vi "CoherenceLength.vi"() -> ()   [LabVIEW 2020]
uses:
  C:/Users/quic2/Desktop/DirectUQDLabviewCode/Kinesis/Thorlabs.MotionControl.Controls.dll
  Kinesis/Thorlabs.MotionControl.Controls.dll
  C:/Program Files/Dotfast Consulting/Timetag Explorer 2.26/ttInterface.dll
  Program Files/Dotfast Consulting/Timetag Explorer 2.26/ttInterface.dll
  C:/Users/quic2/Desktop/DirectUQDLabviewCode/Kinesis/Thorlabs.MotionControl.TCube.StepperMotorCLI.dll
  Kinesis/Thorlabs.MotionControl.TCube.StepperMotorCLI.dll
  <vilib>/Utility/file.llb/Write Delimited Spreadsheet (string).vi
  <vilib>/Utility/file.llb/Write Delimited Spreadsheet (I64).vi
  <vilib>/gmath/statdist.llb/st_Percentiles (scalar).vi
  <vilib>/Utility/file.llb/Write Delimited Spreadsheet (DBL).vi
  <vilib>/gmath/NI_Gmath.lvlib
  <vilib>/Analysis/NI_AALBase.lvlib
panel:
  out "Position":dbl
  out "Pos":i32
  in  "Step(mm)":dbl=0.1
  in  "Stop":dbl=5.5
  in  "Start":dbl=4.5
  in  "TCubeStepperControl":refnum<k24>(container)
  out "XY Graph":cluster{dbl[], dbl[]}[](graph)
  out "BG":dbl[](graph)
  out "bVis":dbl
  out "bMin":dbl
  out "bMax":dbl
  out "Ch C Rate":dbl
  out "Ch C":i32
  out "BG Coincidence Rate":dbl
  out "BG Coincidence":i32
  out "Ch C delay UQD unit":i32
  in  "chC delay":dbl=82.8
  in  "Ch C":i32=8
  in  "stop":bool
  out "sVis":dbl
  out "sMin":dbl
  out "sMax":dbl
  out "cVis":dbl
  out "cMin":dbl
  out "cMax":dbl
  out "Singles":dbl[](graph)
  out "Coincidence":dbl[](graph)
  in  "fileName":string="CTW1ns_ACQ_100ms_Rep_100_ITER_2_Scan_50mHz_6V"
  in  "Folder":path=path "D:/PCC/2021/3_March/20thMarch/SinglePhoton/SourceCharacterisation/CoherenceLength/FinalTestCode"
  out "ChB Delay (uqd Unit)":i32
  out "ChADelay(uqd Unit)":i32
  in  "chB delay (ns)":dbl=7.8
  in  "chA delay(ns)":dbl=110.0
  in  "Ch B":u8=7 min=1 max=16 step=1
  in  "Ch A":u8=5 min=1 max=16 step=1
  in  "CTW in ns":dbl=1.0
  out "Peak Coincidence Rate":dbl format="%#_4p"
  out "ChB Rate":dbl format="%#_4p"
  out "ChARate":dbl format="%#_4p"
  out "Peak Coincidence":i32
  out "Ch A":i32
  out "GetTimeCounter":i32
  out "Ch B":i32
  out "GetResolution":dbl
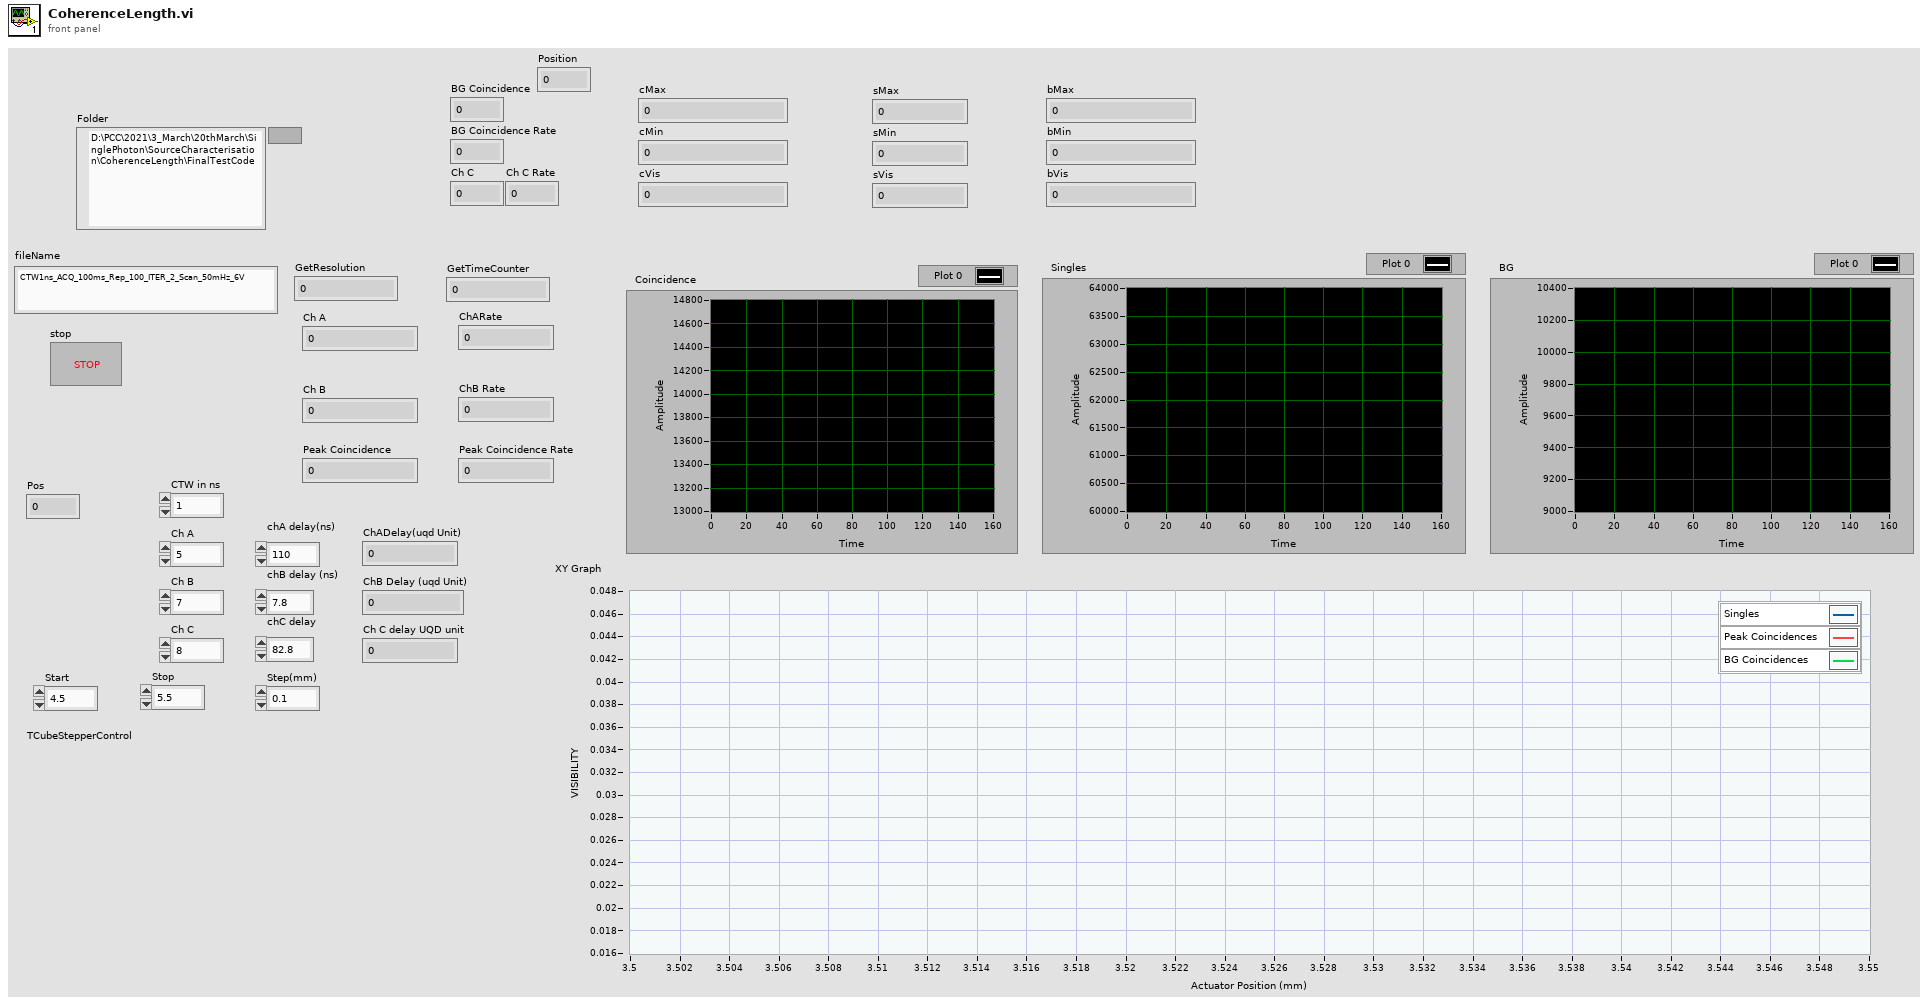
[diagram p1: front panel]
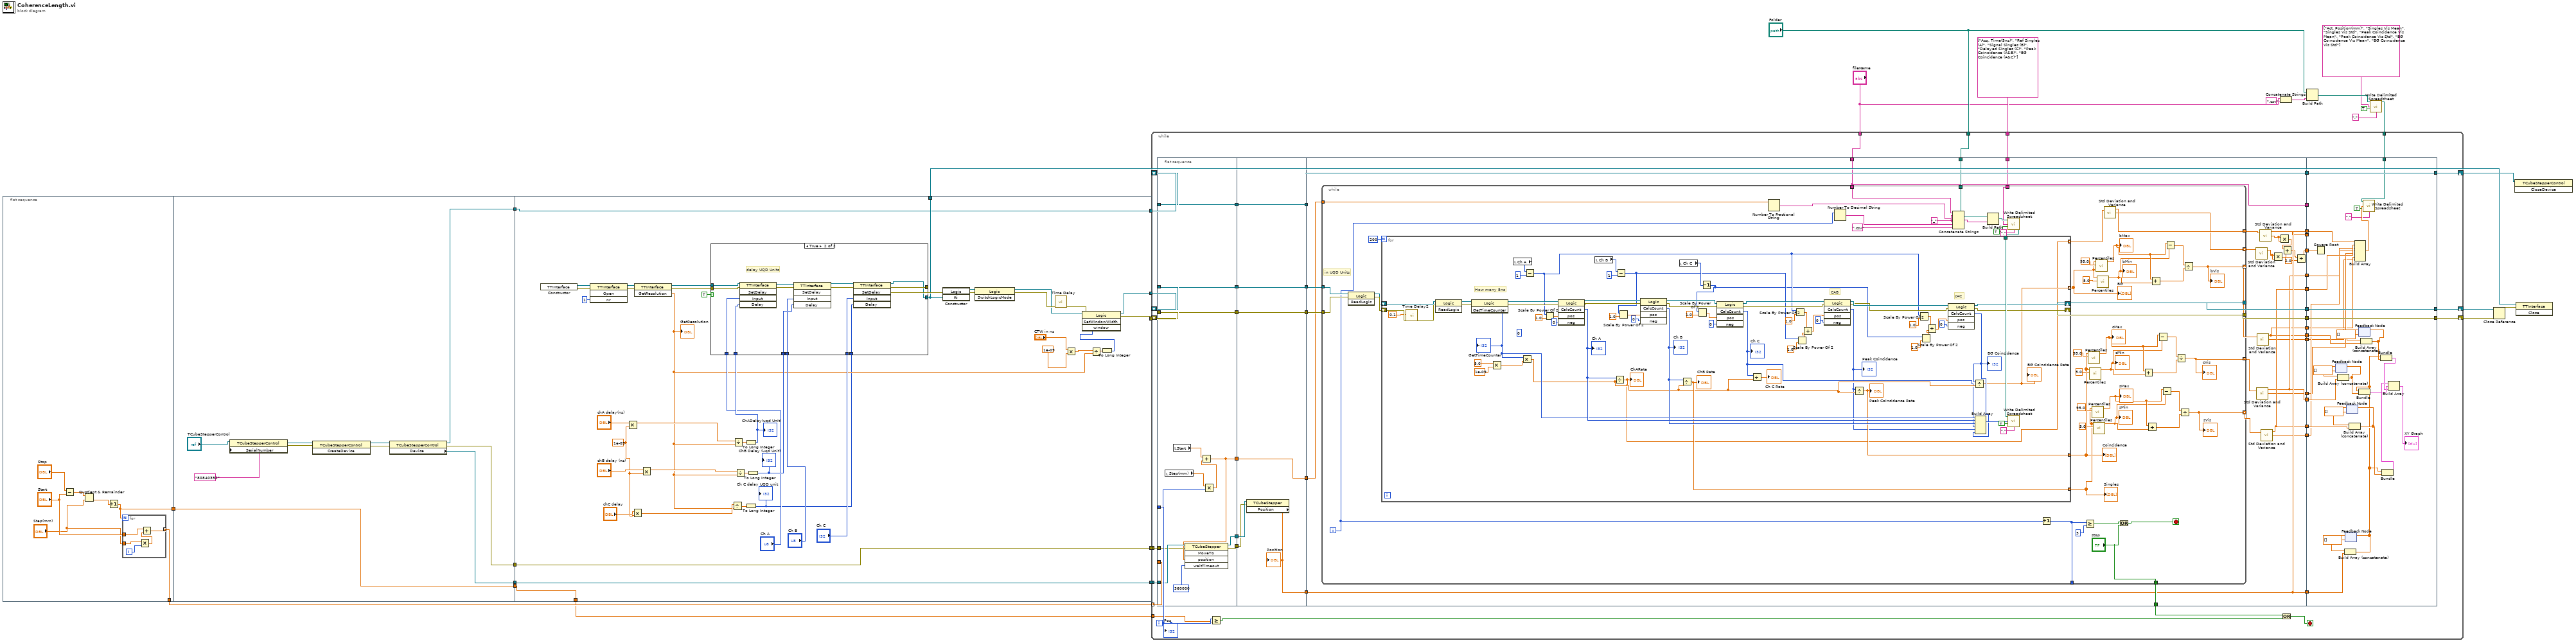
[diagram p0: block diagram]
diagram:
  n1 = flat-sequence {
    tunnel: [w29] -> w14
    tunnel: [w28] -> w11
    tunnel: [w43] -> w21
    tunnel: [w42] -> w20
    tunnel: [w41] -> w16
    tunnel: [w40] -> w12
    tunnel: w11 -> [w40]
    tunnel: [w82] -> w27
    tunnel: [w66] -> w26
    tunnel: [w65] -> w25
    tunnel: w21 -> [w52]
    tunnel: w20 -> [w53]
    tunnel: [w53] -> w19
    tunnel: [w52] -> w17
    tunnel: w16 -> [w51]
    tunnel: [w51] -> w15
    tunnel: [w50] -> w13
    tunnel: w12 -> [w50]
    frame #0 {
      n2 = Subtract(x="Stop", y="Start") -> (x-y=w33:dbl)
      n3 = Quotient & Remainder(x=w33, y="Step(mm)") -> (floor(x/y)=w32:dbl)  [unwired: 1 out]
      n4 = Increment(x=w32) -> (x+1=w28:dbl)
      n5 = for {
        N: w28 -> [_]
        tunnel: "Start" -> [w39]
        tunnel: "Step(mm)" -> [w37]
        tunnel: [w35] -> w29 mode=indexing
        i -> [w38]
        n6 = Multiply(x=w37, y=w38) -> (x*y=w36:dbl)
        n7 = Add(x=w39, y=w36) -> (x+y=w35:dbl)
      }
    }
    frame #1 {
      n8 = property class="TCubeStepperControl"(reference="TCubeStepperControl", "SerialNumber"="80840392") -> (reference out=w46:refnum<k24>, error out=w47:errorcluster)  [unwired: 1 in]
      n9 = invoke class="TCubeStepperControl" method="CreateDevice"(reference=w46, error in=w47) -> (reference out=w45:refnum<k24>, error out=w44:errorcluster)  [unwired: 1 in, 1 out]
      n10 = property class="TCubeStepperControl"(reference=w45, error in=w44) -> (reference out=w42:refnum<k24>, error out=w41:errorcluster, "Device"=w43:refnum<k24>)
    }
    frame #2 {
      w58 = 1e-09
      n11 = constructor class="TTInterface"() -> (reference out=w92:refnum<k24>, error out=w91:errorcluster)  [unwired: 3 in, 1 out]
      n12 = invoke class="TTInterface" method="Open"(reference=w92, error in=w91, "nr"=1) -> (reference out=w88:refnum<k24>, error out=w89:errorcluster)  [unwired: 1 in, 2 out]
      n13 = Multiply(x="chA delay(ns)", y=w58) -> (x*y=w71:dbl)
      n14 = Multiply(x="chC delay", y=w58) -> (x*y=w57:dbl)
      n15 = invoke class="TTInterface" method="GetResolution"(reference=w88, error in=w89) -> (reference out=w87:refnum<k24>, error out=w86:errorcluster, "GetResolution"=w56:dbl)  [unwired: 1 in]
      "GetResolution" <- w56
      n16 = Multiply(x="chB delay (ns)", y=w58) -> (x*y=w70:dbl)
      n17 = Divide(x=w57, y=w56) -> (x/y=w55:dbl)
      n18 = Divide(x=w71, y=w56) -> (x/y=w77:dbl)
      n19 = Divide(x=w70, y=w56) -> (x/y=w76:dbl)
      n20 = To Long Integer(number=w77) -> (32bit integer=w75:i32)
      "ChADelay(uqd Unit)" <- w75
      n21 = To Long Integer(number=w55) -> (32bit integer=w54:i32)
      "Ch C delay UQD unit" <- w54
      n22 = To Long Integer(number=w76) -> (32bit integer=w74:i32)
      "ChB Delay (uqd Unit)" <- w74
      n23 = case shown="True" TRUE {
        tunnel: w87 -> [w94 w108]
        tunnel: w86 -> [w93 w107]
        tunnel: [w93 w97] -> w85
        tunnel: [w94 w98] -> w82
        tunnel: w75 -> [_ w104]
        tunnel: w74 -> [_ w103]
        tunnel: "Ch A" -> [_ w102]
        tunnel: "Ch B" -> [_ w101]
        tunnel: "Ch C" -> [_ w96]
        tunnel: w54 -> [_ w95]
        frame False {
        }
        frame True {
          # "delay UQD Units"
          n24 = invoke class="TTInterface" method="SetDelay"(reference=w108, error in=w107, "Input"=w102, "Delay"=w104) -> (reference out=w106:refnum<k24>, error out=w105:errorcluster)  [unwired: 1 in, 3 out]
          n25 = invoke class="TTInterface" method="SetDelay"(reference=w106, error in=w105, "Input"=w101, "Delay"=w103) -> (reference out=w100:refnum<k24>, error out=w99:errorcluster)  [unwired: 1 in, 3 out]
          n26 = invoke class="TTInterface" method="SetDelay"(reference=w100, error in=w99, "Input"=w96, "Delay"=w95) -> (reference out=w98:refnum<k24>, error out=w97:errorcluster)  [unwired: 1 in, 3 out]
        }
      }
      n27 = constructor class="Logic"(error in=w85, "tti"=w82) -> (reference out=w84:refnum<k24>, error out=w83:errorcluster)  [unwired: 2 in, 2 out]
      n28 = invoke class="Logic" method="SwitchLogicMode"(reference=w84, error in=w83) -> (reference out=w69:refnum<k24>, error out=w81:errorcluster)  [unwired: 1 in, 1 out]
      n29 = call "Time Delay"("error in (no error)"=w81) -> ("error out"=w68:errorcluster)  [unwired: 10 in]
      n30 = Multiply(x="CTW in ns", y=1e-09) -> (x*y=w63:dbl)
      n31 = Divide(x=w63, y=w56) -> (x/y=w62:dbl)
      n32 = To Long Integer(number=w62) -> (32bit integer=w61:i32)
      n33 = invoke class="Logic" method="SetWindowWidth"(reference=w69, error in=w68, "window"=w61) -> (reference out=w66:refnum<k24>, error out=w65:errorcluster)  [unwired: 1 in, 2 out]
    }
  }
  n34 = Concatenate Strings("fileName", ".csv" ("string")) -> (w8:string)
  n35 = Build Path(base path="Folder", name or relative path=w8) -> (appended path=w3:path)
  n36 = call-poly <vilib>:"Write Delimited Spreadsheet.vi"("file path (dialog if empty)"=w3, "1D data"=string[] ["Act. Position(mm)", "Singles Vis Mean", "Singles Vis Std", "Peak Coincidence Vis Mean", "Peak Coincidence Vis Std", "BG Coincidence Vis Mean", "BG Coincidence Vis Std"], "append to file? (new file:F)"=TRUE, "delimiter (\\t)"="," ("delimiter (\\t)")) -> ("new file path (Not A Path if cancelled)"=w2:path)  [unwired: 10 in, 1 out]
  n37 = while {
    shift-right: [w151] -> w23
    shift-left: w26 -> [w154]
    shift-right: [w152] -> w24
    shift-left: w25 -> [w153]
    shift-right: [w149] -> w18
    shift-left: w19 -> [w150]
    tunnel: w17 -> [w148]
    tunnel: w15 -> [w147]
    tunnel: w14 -> [w146] mode=indexing
    tunnel: "Folder" -> [w145]
    tunnel: "fileName" -> [w144]
    tunnel: w13 -> [w129]
    tunnel: string[] ["Acq. Time(5ns)", "Ref Singles (A)", "Signal Singles (B)", "Delayed Singles (C)", "Peak Coincidence (A&B)", "BG Coincidence (A&C)"] -> [w110]
    tunnel: w2 -> [w109]
    i -> [w130]
    stop <- w134 stop-if-true
    n38 = flat-sequence {
      tunnel: w150 -> [w165]
      tunnel: w153 -> [w166]
      tunnel: w154 -> [w167]
      tunnel: [w167] -> w143
      tunnel: [w166] -> w141
      tunnel: [w165] -> w139
      tunnel: w148 -> [w164]
      tunnel: w147 -> [w163]
      tunnel: w130 -> [w157]
      tunnel: w146 -> [_]
      tunnel: [w161] -> w137
      tunnel: [w160] -> w136
      tunnel: [w155] -> w131
      tunnel: w143 -> [w174]
      tunnel: [w174] -> w142
      tunnel: w141 -> [w173]
      tunnel: [w173] -> w140
      tunnel: w139 -> [w172]
      tunnel: [w172] -> w138
      tunnel: w137 -> [w171]
      tunnel: w136 -> [w170]
      tunnel: [w169] -> w135
      tunnel: [w168] -> w132
      tunnel: w131 -> [w168]
      tunnel: w145 -> [w194]
      tunnel: w142 -> [w204]
      tunnel: w140 -> [w203]
      tunnel: w138 -> [w198]
      tunnel: w144 -> [w193]
      tunnel: w135 -> [w192]
      tunnel: [w197] -> w133
      tunnel: w132 -> [w196]
      tunnel: [w202] -> w127
      tunnel: [w201] -> w126
      tunnel: [w198] -> w125
      tunnel: [w192] -> w124
      tunnel: [w181] -> w123
      tunnel: [w179] -> w122
      tunnel: [w177] -> w121
      tunnel: [w193] -> w120
      tunnel: [w192] -> w119
      tunnel: [w190] -> w118
      tunnel: [w184] -> w117
      tunnel: [w181] -> w116
      tunnel: [w180] -> w115
      tunnel: [w179] -> w114
      tunnel: [w178] -> w113
      tunnel: [w177] -> w112
      tunnel: [w176] -> w111
      tunnel: w110 -> [w175]
      tunnel: [w356] -> w149
      tunnel: [w357] -> w151
      tunnel: [w358] -> w152
      tunnel: w127 -> [w358]
      tunnel: w126 -> [w357]
      tunnel: w125 -> [w356]
      tunnel: w124 -> [w355]
      tunnel: w123 -> [w351]
      tunnel: w122 -> [w345]
      tunnel: w121 -> [w339]
      tunnel: w120 -> [_]
      tunnel: w119 -> [w335]
      tunnel: w118 -> [_]
      tunnel: w117 -> [w334]
      tunnel: w116 -> [w333]
      tunnel: w115 -> [w332]
      tunnel: w114 -> [w331]
      tunnel: w113 -> [w330]
      tunnel: w112 -> [w329]
      tunnel: w111 -> [w328]
      tunnel: w109 -> [w324]
      frame #0 {
        n39 = local read "Step(mm)"() -> (w158:dbl)
        n40 = local read "Start"() -> (w159:dbl)
        n41 = Multiply(x=w158, y=w157) -> (x*y=w156:dbl)
        n42 = Add(x=w159, y=w156) -> (x+y=w155:dbl)
        n43 = invoke class="TCubeStepper" method="MoveTo"(reference=w164, error in=w163, "position"=w155, "waitTimeout"=360000) -> (reference out=w161:refnum<k24>, error out=w160:errorcluster)  [unwired: 1 in, 3 out]
      }
      frame #1 {
        n44 = property class="TCubeStepper"(reference=w171, error in=w170) -> ("Position"=w169:dbl)  [unwired: 2 out]
        "Position" <- w169
      }
      frame #2 {
        n45 = while {
          tunnel: w194 -> [w254]
          tunnel: w204 -> [w250]
          tunnel: w203 -> [w249]
          tunnel: [w248] -> w202
          tunnel: [w247] -> w201
          tunnel: [w230] -> _
          tunnel: [w228] -> w200 mode=indexing
          tunnel: [w227] -> w195 mode=indexing
          tunnel: [w220] -> w199 mode=indexing
          tunnel: w193 -> [w218]
          tunnel: w196 -> [w216]
          tunnel: ["stop"] -> w197
          tunnel: [w212] -> w191 mode=indexing
          tunnel: [w211] -> w189 mode=indexing
          tunnel: w175 -> [w205]
          i -> [w232]
          stop <- w214 stop-if-true
          w217 = "_" ("string")
          # "in UQD Units"
          n46 = invoke class="Logic" method="ReadLogic"(reference=w250, error in=w249) -> (reference out=w256:refnum<k24>, error out=w257:errorcluster)  [unwired: 1 in, 1 out]
          n47 = Number To Fractional String(number=w216) -> (F-format string=w215:string)  [unwired: 3 in]
          n48 = Number To Decimal String(number=w232) -> (decimal integer string=w252:string)  [unwired: 1 in]
          n49 = Concatenate Strings(w218, w217, w215, w217, w252, ".csv" ("string")) -> (w253:string)
          n50 = Build Path(base path=w254, name or relative path=w253) -> (appended path=w208:path)
          n51 = call-poly <vilib>:"Write Delimited Spreadsheet.vi"("file path (dialog if empty)"=w208, "1D data"=w205, "append to file? (new file:F)"=TRUE, "delimiter (\\t)"="," ("delimiter (\\t)")) -> ("new file path (Not A Path if cancelled)"=w209:path)  [unwired: 10 in, 1 out]
          n52 = for {
            N: 200 -> [_]
            shift-right: [w270] -> w248
            shift-left: w257 -> [w320]
            shift-right: [w271] -> w247
            shift-left: w256 -> [w319]
            tunnel: w209 -> [w288]
            tunnel: [w287] -> w233 mode=indexing
            tunnel: [w286] -> w245 mode=indexing
            tunnel: [w260] -> w219 mode=indexing
            tunnel: [w259] -> w213 mode=indexing
            (unwired) u8 0 ("y")
            # "cAC"
            # "CAB"
            # "How many 5ns"
            n53 = call "Time Delay2"("error in (no error)"=w320, "Delay Time (s)"=0.1) -> ("error out"=w318:errorcluster)  [unwired: 9 in]
            n54 = invoke class="Logic" method="ReadLogic"(reference=w319, error in=w318) -> (reference out=w313:refnum<k24>, error out=w312:errorcluster)  [unwired: 1 in, 1 out]
            n55 = invoke class="Logic" method="GetTimeCounter"(reference=w313, error in=w312) -> (reference out=w308:refnum<k24>, error out=w307:errorcluster, "GetTimeCounter"=w291:i32)  [unwired: 1 in]
            "GetTimeCounter" <- w291
            n56 = Multiply(x=5.0, y=1e-09) -> (x*y=w314:dbl)
            n57 = local read "Ch A"() -> (w298:u8)
            n58 = Multiply(x=w291, y=w314) -> (x*y=w265:dbl)
            n59 = Subtract(x=w298, y=u8 1) -> (x-y=w267:u8)
            n60 = Scale By Power Of 2(n=w267, x=1.0) -> (x*2^n=w310:dbl)
            n61 = invoke class="Logic" method="CalcCount"(reference=w308, error in=w307, "pos"=w310, "neg"=0) -> (reference out=w306:refnum<k24>, error out=w305:errorcluster, "CalcCount"=w294:i32)  [unwired: 1 in, 2 out]
            "Ch A" <- w294
            n62 = local read "Ch B"() -> (w296:u8)
            n63 = Divide(x=w294, y=w265) -> (x/y=w259:dbl)
            "ChARate" <- w259
            n64 = Subtract(x=w296, y=u8 1) -> (x-y=w266:u8)
            n65 = Scale By Power Of 2(n=w266, x=1.0) -> (x*2^n=w322:dbl)
            n66 = invoke class="Logic" method="CalcCount"(reference=w306, error in=w305, "pos"=w322, "neg"=0) -> (reference out=w285:refnum<k24>, error out=w284:errorcluster, "CalcCount"=w293:i32)  [unwired: 1 in, 2 out]
            "Ch B" <- w293
            n67 = local read "Ch C"() -> (w278:i32)
            n68 = Divide(x=w293, y=w265) -> (x/y=w287:dbl)
            "ChB Rate" <- w287
            n69 = Decrement(x=w278) -> (x-1=w258:i32)
            n70 = Scale By Power Of 2(n=w258, x=1.0) -> (x*2^n=w280:dbl)
            n71 = invoke class="Logic" method="CalcCount"(reference=w285, error in=w284, "pos"=w280, "neg"=0) -> (reference out=w283:refnum<k24>, error out=w282:errorcluster, "CalcCount"=w263:i32)  [unwired: 1 in, 2 out]
            "Ch C" <- w263
            n72 = Divide(x=w263, y=w265) -> (x/y=→"Ch C Rate":dbl)
            n73 = Scale By Power Of 2(n=w267, x=1.0) -> (x*2^n=w301:dbl)
            n74 = Scale By Power Of 2(n=w266, x=1.0) -> (x*2^n=w300:dbl)
            n75 = Add(x=w301, y=w300) -> (x+y=w299:dbl)
            n76 = invoke class="Logic" method="CalcCount"(reference=w283, error in=w282, "pos"=w299, "neg"=0) -> (reference out=w269:refnum<k24>, error out=w268:errorcluster, "CalcCount"=w262:i32)  [unwired: 1 in, 2 out]
            "Peak Coincidence" <- w262
            n77 = Divide(x=w262, y=w265) -> (x/y=w286:dbl)
            "Peak Coincidence Rate" <- w286
            n78 = Scale By Power Of 2(n=w267, x=1.0) -> (x*2^n=w274:dbl)
            n79 = Scale By Power Of 2(n=w258, x=1.0) -> (x*2^n=w273:dbl)
            n80 = Add(x=w274, y=w273) -> (x+y=w272:dbl)
            n81 = invoke class="Logic" method="CalcCount"(reference=w269, error in=w268, "pos"=w272, "neg"=0) -> (reference out=w271:refnum<k24>, error out=w270:errorcluster, "CalcCount"=w261:i32)  [unwired: 1 in, 2 out]
            "BG Coincidence" <- w261
            n82 = Divide(x=w261, y=w265) -> (x/y=w260:dbl)
            "BG Coincidence Rate" <- w260
            n83 = Build Array(w291, w294, w293, w263, w262, w261) -> (w292:i32[])
            n84 = call-poly <vilib>:"Write Delimited Spreadsheet.vi"("file path (dialog if empty)"=w288, "1D data"=w292, "append to file? (new file:F)"=TRUE, "delimiter (\\t)"="," ("delimiter (\\t)")) -> ()  [unwired: 10 in, 2 out]
          }
          "Coincidence" <- w245
          "Singles" <- w233
          "BG" <- w219
          n85 = Increment(x=w232) -> (x+1=w230:i32)
          n86 = Greater Or Equal?(x=w230, y=3) -> (x >= y?=w229:bool)
          n87 = call-poly <vilib>:"Percentiles.vi"("p"=95.0, "x array"=w245) -> ("percentile"=w242:dbl)  [unwired: 8 in, 1 out]
          "cMax" <- w242
          n88 = call-poly <vilib>:"Percentiles.vi"("p"=5.0, "x array"=w245) -> ("percentile"=w241:dbl)  [unwired: 8 in, 1 out]
          "cMin" <- w241
          n89 = call-poly <vilib>:"Percentiles.vi"("p"=95.0, "x array"=w233) -> ("percentile"=w236:dbl)  [unwired: 8 in, 1 out]
          "sMax" <- w236
          n90 = call-poly <vilib>:"Percentiles.vi"("p"=5.0, "x array"=w233) -> ("percentile"=w235:dbl)  [unwired: 8 in, 1 out]
          "sMin" <- w235
          n91 = call-poly <vilib>:"Percentiles.vi"("p"=95.0, "x array"=w219) -> ("percentile"=w223:dbl)  [unwired: 8 in, 1 out]
          "bMax" <- w223
          n92 = call-poly <vilib>:"Percentiles.vi"("p"=5.0, "x array"=w219) -> ("percentile"=w222:dbl)  [unwired: 8 in, 1 out]
          "bMin" <- w222
          n93 = call <vilib>:"Std Deviation and Variance.vi"("X"=w213) -> ("mean"=w212:dbl, "standard deviation"=w211:dbl)  [unwired: 1 in, 1 out]
          n94 = Or(x=w229, y="stop") -> (x .or. y?=w214:bool)
          n95 = Add(x=w242, y=w241) -> (x+y=w240:dbl)
          n96 = Add(x=w236, y=w235) -> (x+y=w234:dbl)
          n97 = Add(x=w223, y=w222) -> (x+y=w221:dbl)
          n98 = Subtract(x=w242, y=w241) -> (x-y=w243:dbl)
          n99 = Subtract(x=w236, y=w235) -> (x-y=w237:dbl)
          n100 = Subtract(x=w223, y=w222) -> (x-y=w224:dbl)
          n101 = Divide(x=w243, y=w240) -> (x/y=w228:dbl)
          "cVis" <- w228
          n102 = Divide(x=w237, y=w234) -> (x/y=w227:dbl)
          "sVis" <- w227
          n103 = Divide(x=w224, y=w221) -> (x/y=w220:dbl)
          "bVis" <- w220
        }
        n104 = call <vilib>:"Std Deviation and Variance.vi"("X"=w189) -> ("mean"=w187:dbl)  [unwired: 1 in, 2 out]
        n105 = call <vilib>:"Std Deviation and Variance.vi"("X"=w200) -> ("mean"=w179:dbl, "standard deviation"=w178:dbl)  [unwired: 1 in, 1 out]
        n106 = call <vilib>:"Std Deviation and Variance.vi"("X"=w199) -> ("mean"=w177:dbl, "standard deviation"=w176:dbl)  [unwired: 1 in, 1 out]
        n107 = call <vilib>:"Std Deviation and Variance.vi"("X"=w191) -> ("mean"=w190:dbl, "standard deviation"=w188:dbl)  [unwired: 1 in, 1 out]
        n108 = call <vilib>:"Std Deviation and Variance.vi"("X"=w195) -> ("mean"=w181:dbl, "standard deviation"=w180:dbl)  [unwired: 1 in, 1 out]
        n109 = Multiply(x=w187, y=w187) -> (x*y=w186:dbl)
        n110 = Multiply(x=w188, y=w188) -> (x*y=w185:dbl)
        n111 = Add(x=w185, y=w186) -> (x+y=w183:dbl)
        n112 = Divide(x=w183, y=2.0) -> (x/y=w184:dbl)
      }
      frame #3 {
        n113 = Square Root(x=w334) -> ()  [unwired: 1 out]
        n114 = feedback #1(dbl[] []) -> (w346:dbl[])
        n115 = Build Array (concatenate)(w346, w345) -> (w343:dbl[])
        n116 = feedback-in #1(w343) -> ()
        n117 = feedback #2(dbl[] []) -> (w354:dbl[])
        n118 = Build Array (concatenate)(w354, w355) -> (w337:dbl[])
        n119 = feedback-in #2(w337) -> ()
        n120 = feedback #3(dbl[] []) -> (w352:dbl[])
        n121 = Build Array (concatenate)(w352, w351) -> (w349:dbl[])
        n122 = feedback-in #3(w349) -> ()
        n123 = Build Array(w335, w333, w332, w331, w330, w329, w328) -> (w327:dbl[])
        n124 = feedback #4(dbl[] []) -> (w341:dbl[])
        n125 = Bundle(w337, w343) -> (w342:cluster{dbl[], dbl[]})  [unwired: 1 in]
        n126 = Build Array (concatenate)(w341, w339) -> (w338:dbl[])
        n127 = feedback-in #4(w338) -> ()
        n128 = call-poly <vilib>:"Write Delimited Spreadsheet.vi"("file path (dialog if empty)"=w324, "1D data"=w327, "append to file? (new file:F)"=TRUE, "delimiter (\\t)"="," ("delimiter (\\t)")) -> ()  [unwired: 10 in, 2 out]
        n129 = Bundle(w337, w338) -> (w336:cluster{dbl[], dbl[]})  [unwired: 1 in]
        n130 = Bundle(w337, w349) -> (w348:cluster{dbl[], dbl[]})  [unwired: 1 in]
        n131 = Build Array(w348, w342, w336) -> (→"XY Graph":cluster{dbl[], dbl[]}[])
      }
    }
    n132 = Greater Or Equal?(x=w130, y=w129) -> (x >= y?=w128:bool)
    n133 = Or(x=w133, y=w128) -> (x .or. y?=w134:bool)
    "Pos" <- w130
  }
  n134 = Close Reference(reference=w23, error in (no error)=w24) -> (error out=w22:errorcluster)
  n135 = invoke class="TCubeStepperControl" method="CloseDevice"(reference=w18) -> ()  [unwired: 2 in, 3 out]
  n136 = invoke class="TTInterface" method="Close"(reference=w27, error in=w22) -> ()  [unwired: 1 in, 3 out]
